vi "Change_Sample_Rate.vi"(2 "error in":errorcluster, 3 "Period (ms)":u32, 4 "Device Session In":refnum<visa-resource-name>) -> (0 "error out":errorcluster, 1 "Device Session Out":refnum<visa-resource-name>)   [LabVIEW 2017]
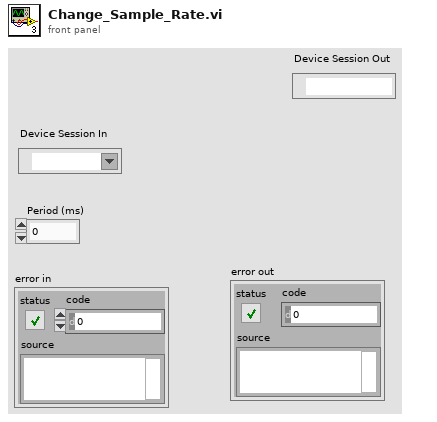
[diagram p1: front panel]
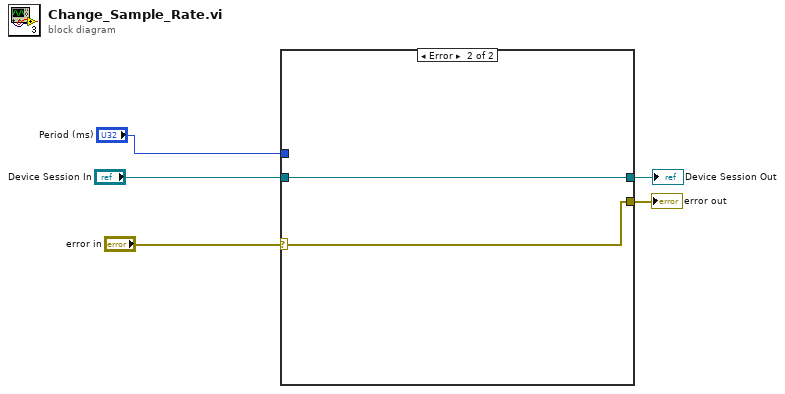
[diagram p0: block diagram]
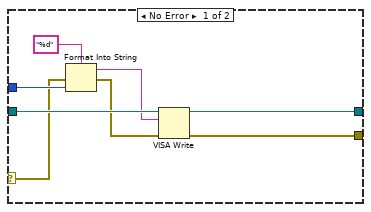
[diagram p2: hidden frame]
diagram:
  n1 = case shown="Error" "error in" {
    selector: "error in" -> [w6 w14]
    tunnel: "Device Session In" -> [w13 w15]
    tunnel: "Period (ms)" -> [w11 _]
    tunnel: [w9 w14] -> w2
    tunnel: [w8 w15] -> w1
    frame No Error {
      n2 = Format Into String(format string="%d", error in=w6, w11) -> (resulting string=w10:string, error out=w7:errorcluster)  [unwired: 1 in]
      n3 = VISA Write(VISA resource name=w13, write buffer=w10, error in (no error)=w7) -> (VISA resource name out=w8:refnum<visa-resource-name>, error out=w9:errorcluster)  [unwired: 1 out]
    }
    frame Error {
    }
  }
  "error out" <- w2
  "Device Session Out" <- w1
